vi "Pacman2018.vi"() -> ()   [LabVIEW 2018]
uses:
  AD14/Debug/EasyDLL.dll
panel:
  in  "Scopul jocului : trebuie sa ajungi in coltul cel mai din dreapta-jos, fara sa te prinda cei doi inamici.\n      Mod de joc : butonul START initializeaza harta\nsi sagetile muta jucatorul.":bool
  out "Tabla de joc":bool[][](array[boolean])
  out "Coordonate\n            Jucator                     Obstacol1                 Obstacol2 2":i32[](array[numeric])
  out "Starea jocului":string
  in  "Up":bool
  in  "Right":bool
  in  "Left":bool
  in  "Down":bool
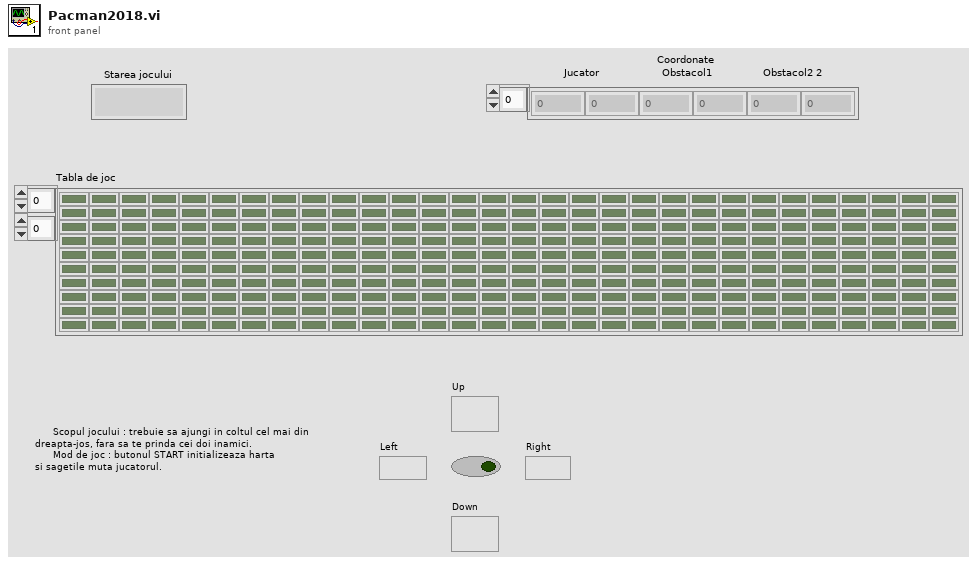
[diagram p1: front panel]
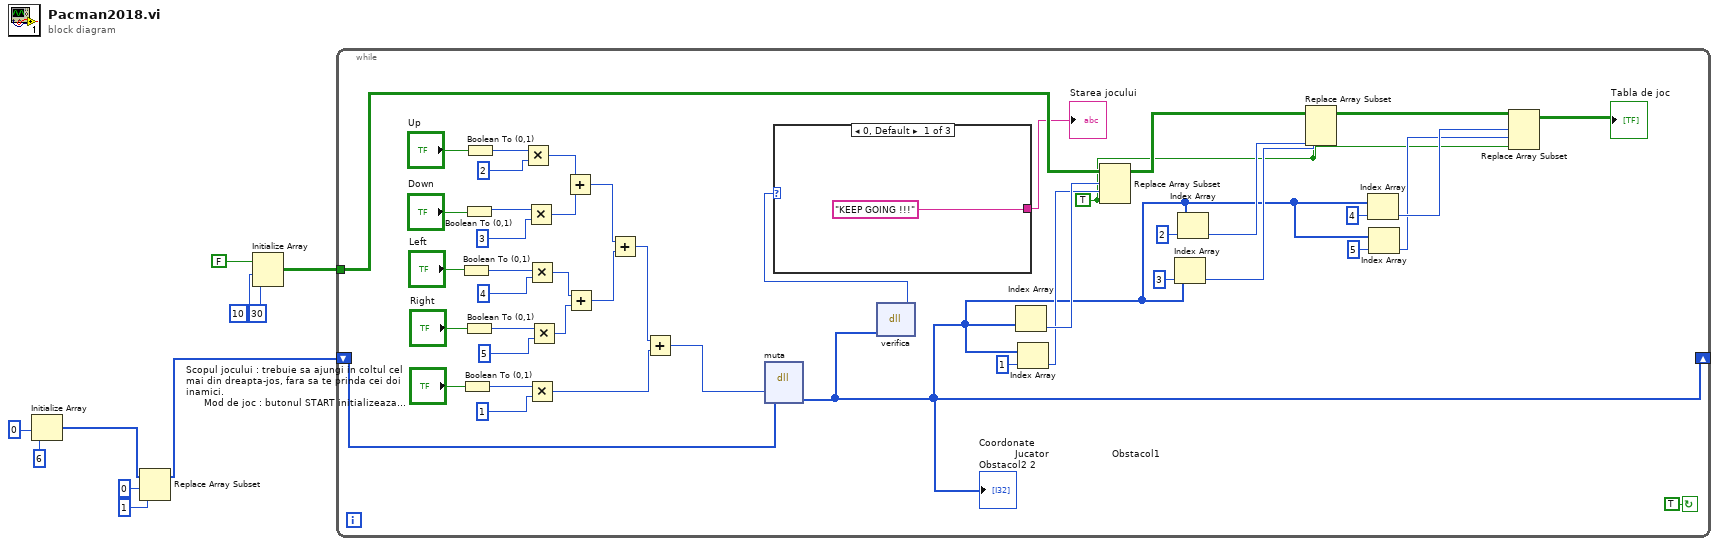
[diagram p0: block diagram]
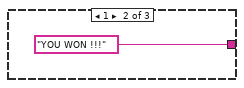
[diagram p2: hidden frame]
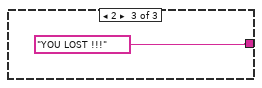
[diagram p3: hidden frame]
diagram:
  n1 = Initialize Array(0, 6) -> (w3:i32[])
  n2 = Replace Array Subset(array=w3, new element=1 ("new element/subarray"), index=0) -> (w4:i32[])
  n3 = Initialize Array(FALSE ("Boolean"), 10 ("dimension size"), 30 ("dimension size")) -> (w5:bool[][])
  n4 = while {
    shift-right: [w17] -> _
    shift-left: w4 -> [w55]
    tunnel: w5 -> [w34]
    stop <- TRUE continue-if-true
    w14 = TRUE ("new element/subarray")
    n5 = Boolean To (0,1)(Boolean="Left") -> (0, 1=w47:i16)
    n6 = Boolean To (0,1)(Boolean="Scopul jocului : trebuie sa ajungi in coltul cel mai din dreapta-jos, fara sa te prinda cei doi inamici.\n      Mod de joc : butonul START initializeaza harta\nsi sagetile muta jucatorul.") -> (0, 1=w31:i16)
    n7 = Boolean To (0,1)(Boolean="Down") -> (0, 1=w49:i16)
    n8 = Boolean To (0,1)(Boolean="Right") -> (0, 1=w48:i16)
    n9 = Boolean To (0,1)(Boolean="Up") -> (0, 1=w43:i16)
    n10 = Multiply(x=w43, y=2) -> (x*y=w51:i32)
    n11 = Multiply(x=w49, y=3) -> (x*y=w50:i32)
    n12 = Multiply(x=w47, y=4) -> (x*y=w53:i32)
    n13 = Multiply(x=w31, y=1) -> (x*y=w28:i32)
    n14 = Multiply(x=w48, y=5) -> (x*y=w52:i32)
    n15 = Add(x=w51, y=w50) -> (x+y=w37:i32)
    n16 = Add(x=w53, y=w52) -> (x+y=w36:i32)
    n17 = Add(x=w37, y=w36) -> (x+y=w29:i32)
    n18 = Add(x=w29, y=w28) -> (x+y=w27:i32)
    n19 = dll-call lib="C:/Users/danyr/OneDrive/Desktop/ProiectFinalAD/AD14/Debug/EasyDLL.dll" fn="muta"("arg1"=w27, "arg2"=w55) -> ("arg2"=w17:i32[])  [unwired: 5 in, 2 out]
    "Coordonate\n            Jucator                     Obstacol1                 Obstacol2 2" <- w17
    n20 = dll-call lib="C:/Users/danyr/OneDrive/Desktop/ProiectFinalAD/AD14/Debug/EasyDLL.dll" fn="verifica"("arg1"=w17) -> ("return type"=w54:i32)  [unwired: 4 in, 2 out]
    n21 = case shown="0, Default" w54 {
      tunnel: ["KEEP GOING !!!" "YOU WON !!!" "YOU LOST !!!"] -> w26
      frame 0, Default {
      }
      frame 1 {
      }
      frame 2 {
      }
    }
    "Starea jocului" <- w26
    n22 = Index Array(array=w17) -> (element=w33:i32)  [unwired: 1 in]
    n23 = Index Array(array=w17, index=1) -> (element=w32:i32)
    n24 = Replace Array Subset(array=w34, new element=w14, index (row)=w33, index (col)=w32) -> (w21:bool[][])
    n25 = Index Array(array=w17, index=3) -> (element=w22:i32)
    n26 = Index Array(array=w17, index=2) -> (element=w23:i32)
    n27 = Replace Array Subset(array=w21, new element=w14, index (row)=w23, index (col)=w22) -> (w20:bool[][])
    n28 = Index Array(array=w17, index=4) -> (element=w16:i32)
    n29 = Index Array(array=w17, index=5) -> (element=w15:i32)
    n30 = Replace Array Subset(array=w20, new element=w14, index (row)=w16, index (col)=w15) -> (→"Tabla de joc":bool[][])
  }
